vi "TrajectoryGenerate_Make_Quintic_Weighted.vi"(8 "traj_config":T7 {"End Velocity" format="%20.4f"; "StartVelocity" format="%20.4f"; "Max Acceleration" format="%20.4f"; "MaxVelocity" format="%20.4f"}, 11 "WeightedWaypointPOSE":T1[](array[typedef]) {"SCALAR" format="%14.3f"; "ROTATION"."SIN" format="%13.4f"; "ROTATION"."COS" format="%13.4f"; "ROTATION"."VALUE" format="%13.4f"; "TRANSLATION"."Y" format="%14.3f"; "TRANSLATION"."X" format="%14.3f"}) -> (0 "error out":errorcluster, 3 "TRAJECTORY":T4 {"States"."POSE"."ROTATION"."SIN" format="%13.4f"; "States"."POSE"."ROTATION"."COS" format="%13.4f"; "States"."POSE"."ROTATION"."VALUE" format="%13.4f"; "States"."POSE"."TRANSLATION"."Y" format="%14.3f"; "States"."POSE"."TRANSLATION"."X" format="%14.3f"; "TotalTImeSecs" format="%20.3f"})   [LabVIEW 2019, in "Trajectory_Library.lvlib"]
doc: "Generates a trajectory from the given weighted waypoints and config. This method uses quintic hermite splines -- therefore, all points must be represented by Pose2d objects. Continuous curvature is guaranteed in this method.\n\nParameters:\n - WeightedWaypointPose - Array of weighted waypoints .\n - Trajectory Config - The configuration for the trajectory.\n\nReturns:\n - Trajectory -- Created trajectory data structure\n - Error Out - Returned error cluster"
uses:
  Trajectory_Library.lvlib
  TypeDef/TRAJ_CONFIG.ctl
  TypeDef/TRAJECTORY.ctl
  TypeDef/TRAJ_STATE.ctl
  TypeDef/POSE2D.ctl
  TypeDef/TRANSLATION2D.ctl
  TypeDef/ROTATION2D.ctl
  TypeDef/WEIGHTED_WAYPOINT.ctl
  TypeDef/POSEwCURVATURE.ctl
  Conv_Deg_Radians.vi
  Rotation2d_CreateAngle.vi
  Pose2d_TransformBy.vi
  Translation2d_RotateBy.vi
  Translation2d_Plus.vi
  Rotation2d_Plus.vi
  Rotation2d_RotateBy.vi
  Rotation2d_CreateXY.vi
  Util_CalcDist.vi
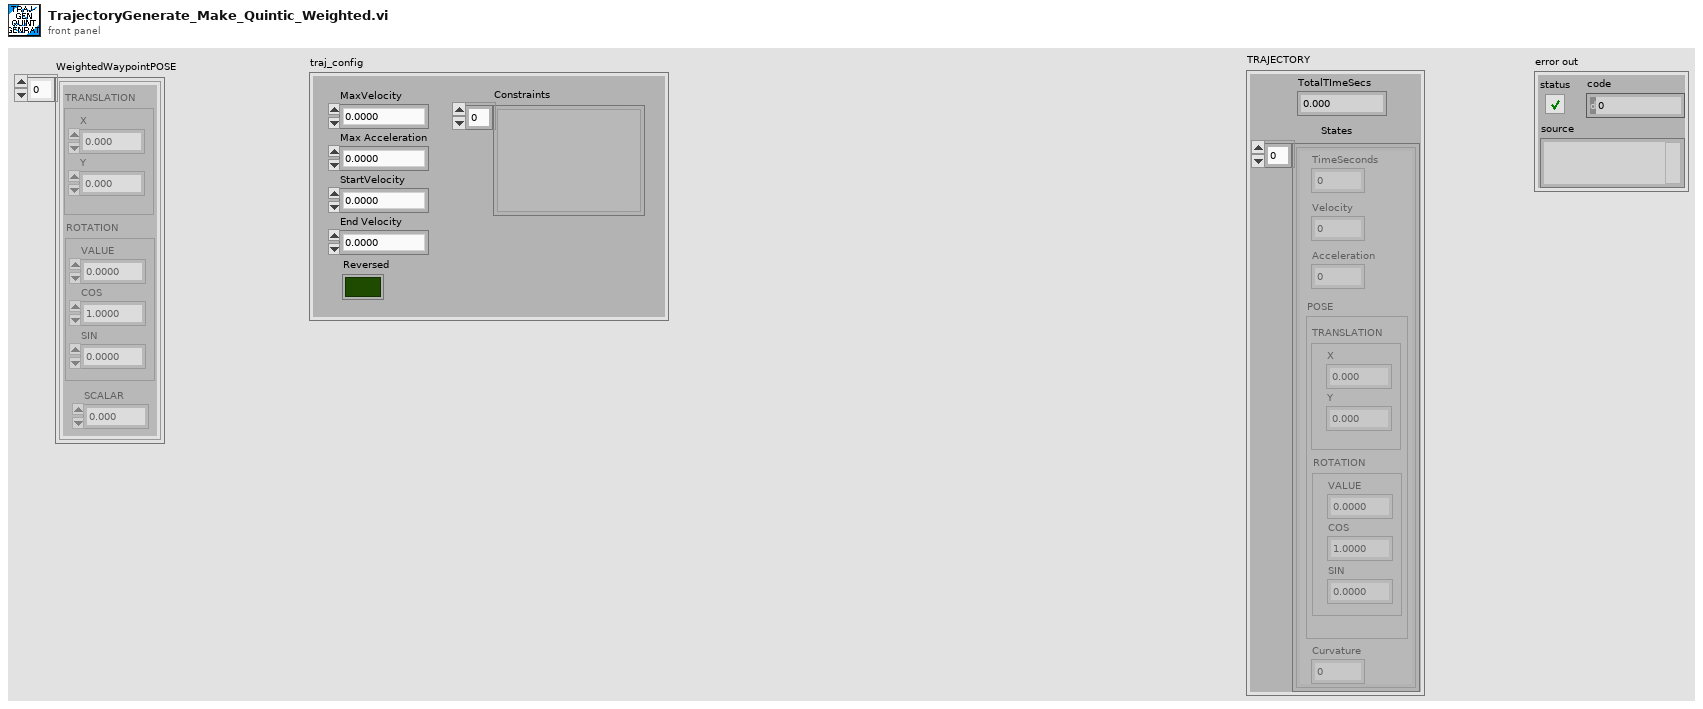
[diagram p1: front panel]
types:
  T1 = typedef "Trajectory_Library.lvlib/WEIGHTED_WAYPOINT.ctl" = cluster{"TRANSLATION":T2, "ROTATION":T3, "SCALAR":dbl}
  T2 = typedef "Trajectory_Library.lvlib/TRANSLATION2D.ctl" = cluster{"X":dbl, "Y":dbl}
  T3 = typedef "Trajectory_Library.lvlib/ROTATION2D.ctl" = cluster{"VALUE":dbl, "COS":dbl, "SIN":dbl}
  T4 = typedef "Trajectory_Library.lvlib/TRAJECTORY.ctl" = cluster{"TotalTImeSecs":dbl, "States":T5[]}
  T5 = typedef "Trajectory_Library.lvlib/TRAJ_STATE.ctl" = cluster{"TimeSeconds":dbl, "Velocity":dbl, "Acceleration":dbl, "POSE":T6, "Curvature":dbl}
  T6 = typedef "Trajectory_Library.lvlib/POSE2D.ctl" = cluster{"TRANSLATION":T2, "ROTATION":T3}
  T7 = typedef "Trajectory_Library.lvlib/TRAJ_CONFIG.ctl" = cluster{"MaxVelocity":dbl, "Max Acceleration":dbl, "StartVelocity":dbl, "End Velocity":dbl, "Reversed":bool, "Constraints":variant[]}
  T8 = typedef "Trajectory_Library.lvlib/TRANSFORM2D.ctl" = cluster{"TRANSLATION":T2, "ROTATION":T3, "xF":bool}
  T9 = typedef "Trajectory_Library.lvlib/SPLINE.ctl" = cluster{"Degree":i32, "Coefficients":T10}
  T10 = typedef "NI_Matrix.lvlib/RealMatrix.ctl" = dbl[][]
  T11 = typedef "Trajectory_Library.lvlib/POSEwCURVATURE.ctl" = cluster{"CURVATURE":dbl, "POSE":T6}
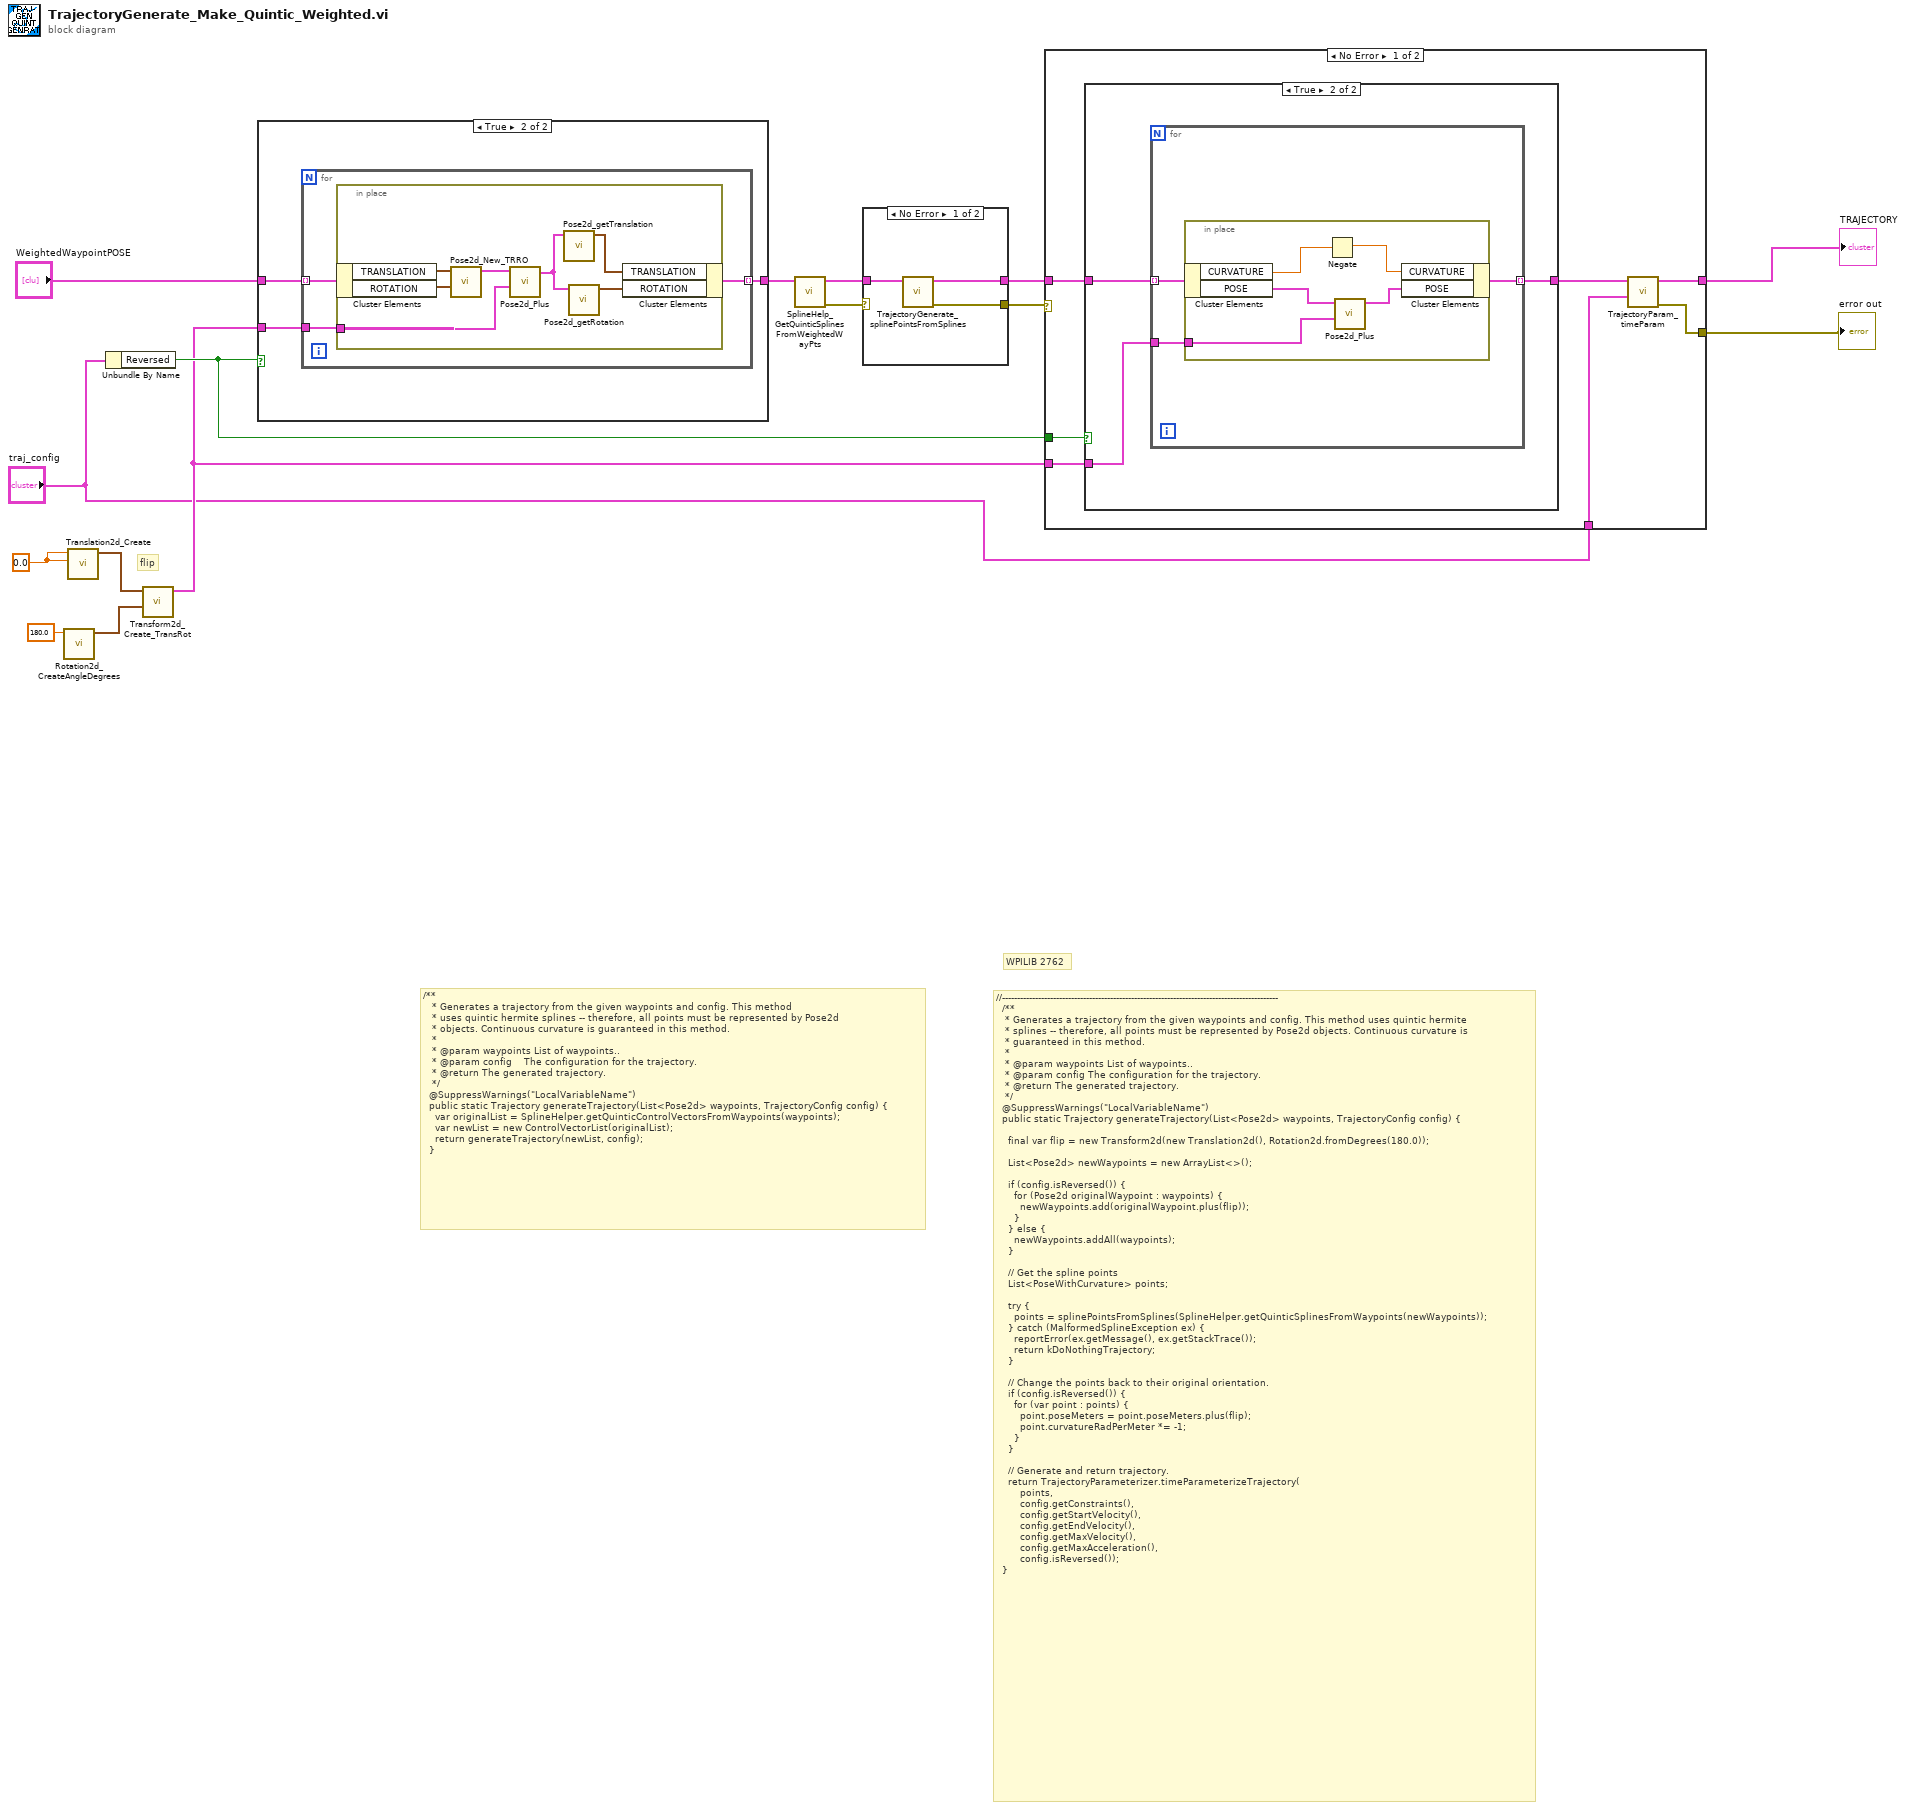
[diagram p0: block diagram]
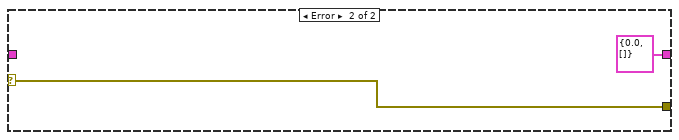
[diagram p3: hidden frame]
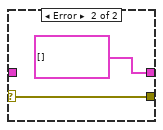
[diagram p4: hidden frame]
diagram:
  w13 = 0.0 ("X")
  # "flip"
  # "WPILIB 2762"
  # "//--------------------------------------------------------------------------------------------\n  /**\n   * Generates a trajectory from the given waypoints and config. This method uses quintic hermite\n   * splines -- therefore, all points must be represented by Pose2d objects. Continuous curvature is\n   * guaranteed in this method.\n   *\n   * @param waypoints List of waypoints..\n   * @param config The configuration for the trajectory.\n   * @return The generated trajectory.\n   */\n  @SuppressWarnings(\"LocalVariableName\")\n  public static Trajectory generateTrajectory(List<Pose2d> waypoints, TrajectoryConfig config) {\n\n    final var flip = new Transform2d(new Translation2d(), Rotation2d.fromDegrees(180.0));\n\n    List<Pose2d> newWaypoints = new ArrayList<>();\n\n    if (config.isReversed()) {\n      for (Pose2d originalWaypoint : waypoints) {\n        newWaypoints.add(originalWaypoint.plus(flip));\n      }\n    } else {\n      newWaypoints.addAll(waypoints);\n    }\n\n    // Get the spline points\n    List<PoseWithCurvature> points;\n\n    try {\n      points = splinePointsFromSplines(SplineHelper.getQuinticSplinesFromWaypoints(newWaypoints));\n    } catch (MalformedSplineException ex) {\n      reportError(ex.getMessage(), ex.getStackTrace());\n      return kDoNothingTrajectory;\n    }\n\n    // Change the points back to their original orientation.\n    if (config.isReversed()) {\n      for (var point : points) {\n        point.poseMeters = point.poseMeters.plus(flip);\n        point.curvatureRadPerMeter *= -1;\n      }\n    }\n\n    // Generate and return trajectory.\n    return TrajectoryParameterizer.timeParameterizeTrajectory(\n        points,\n        config.getConstraints(),\n        config.getStartVelocity(),\n        config.getEndVelocity(),\n        config.getMaxVelocity(),\n        config.getMaxAcceleration(),\n        config.isReversed());\n  }"
  # "/**\n   * Generates a trajectory from the given waypoints and config. This method\n   * uses quintic hermite splines -- therefore, all points must be represented by Pose2d\n   * objects. Continuous curvature is guaranteed in this method.\n   *\n   * @param waypoints List of waypoints..\n   * @param config    The configuration for the trajectory.\n   * @return The generated trajectory.\n   */\n  @SuppressWarnings(\"LocalVariableName\")\n  public static Trajectory generateTrajectory(List<Pose2d> waypoints, TrajectoryConfig config) {\n    var originalList = SplineHelper.getQuinticControlVectorsFromWaypoints(waypoints);\n    var newList = new ControlVectorList(originalList);\n    return generateTrajectory(newList, config);\n  }"
  n1 = call "Rotation2d_CreateAngleDegrees.vi"("Angle_Degrees"=180.0) -> ("ROTATION"=w15:T3)  [unwired: 10 in]
  n2 = call "Translation2d_Create.vi"("Y"=w13, "X"=w13) -> ("TRANSLATION"=w12:T2)  [unwired: 9 in]
  n3 = Unbundle By Name("traj_config") -> ("Reversed"=w6:bool)
  n4 = call "Transform2d_Create_TransRot.vi"("ROTATION"=w15, "TRANSLATION"=w12) -> ("TRANSFORM"=w4:T8)  [unwired: 9 in]
  n5 = case shown="True" w6 {
    tunnel: "WeightedWaypointPOSE" -> [w16 w19]
    tunnel: w4 -> [_ w18]
    tunnel: [w16 w17] -> w10
    frame False {
    }
    frame True {
      n6 = for {
        tunnel: w19 -> [w21] mode=indexing
        tunnel: w18 -> [w22]
        tunnel: [w20] -> w17 mode=indexing
        n7 = in-place {
          in-place-border: w22 -> [w26]
          n8 = in-place-cluster #1(w21) -> ("TRANSLATION"=w29:T2, "ROTATION"=w28:T3)
          n9 = call "Pose2d_New_TRRO.vi"("ROTATION"=w28, "TRANSLATION"=w29) -> ("outPOSE"=w27:T6)  [unwired: 9 in]
          n10 = call "Pose2d_Plus.vi"("other TRANSFORM"=w26, "in POSE"=w27) -> ("out POSE"=w23:T6)  [unwired: 9 in]
          n11 = call "Pose2d_getTranslation.vi"("in POSE"=w23) -> ("outTRANSLATION"=w24:T2)  [unwired: 10 in]
          n12 = call "Pose2d_getRotation.vi"("in POSE"=w23) -> ("out ROTATION"=w25:T3)  [unwired: 10 in]
          n13 = in-place-cluster #1("TRANSLATION"=w24, "ROTATION"=w25) -> (w20:T1)
        }
      }
    }
  }
  n14 = call "SplineHelp_GetQuinticSplinesFromWeightedWayPts.vi"("WeightedWayPoints"=w10) -> ("out Error"=w9:errorcluster, "Splines"=w8:T9[])  [unwired: 9 in]
  n15 = case shown="No Error" w9 {
    selector: w9 -> [_ w34]
    tunnel: w8 -> [w32 _]
    tunnel: [w31 w34] -> w7
    tunnel: [w30 T11[] [] ("ArrayPoseWithCurvature")] -> w5
    frame No Error {
      n16 = call "TrajectoryGenerate_splinePointsFromSplines.vi"("inputSPLINE"=w32) -> ("error out"=w31:errorcluster, "ArrayPoseWithCurvature"=w30:T11[])  [unwired: 9 in]
    }
    frame Error {
    }
  }
  n17 = case shown="No Error" w7 {
    selector: w7 -> [_ w55]
    tunnel: w6 -> [w41 _]
    tunnel: w5 -> [w40 _]
    tunnel: w4 -> [w39 _]
    tunnel: "traj_config" -> [w37 _]
    tunnel: [w36 T4 {"TotalTImeSecs"=0.0, "States"=[]} ("TRAJECTORY")] -> w2
    tunnel: [w35 w55] -> w1
    frame No Error {
      n18 = case shown="True" w41 {
        tunnel: w40 -> [w42 w45]
        tunnel: w39 -> [_ w44]
        tunnel: [w42 w43] -> w38
        frame False {
        }
        frame True {
          n19 = for {
            tunnel: w45 -> [w48] mode=indexing
            tunnel: w44 -> [w47]
            tunnel: [w46] -> w43 mode=indexing
            n20 = in-place {
              in-place-border: w47 -> [w49]
              n21 = in-place-cluster #2(w48) -> ("CURVATURE"=w53:dbl, "POSE"=w52:T6)
              n22 = Negate(x=w53) -> (-x=w50:dbl)
              n23 = call "Pose2d_Plus.vi"("other TRANSFORM"=w49, "in POSE"=w52) -> ("out POSE"=w51:T6)  [unwired: 9 in]
              n24 = in-place-cluster #2("CURVATURE"=w50, "POSE"=w51) -> (w46:T11)
            }
          }
        }
      }
      n25 = call "TrajectoryParam_timeParam.vi"("TRAJECTORY_CONFIG"=w37, "points"=w38) -> ("error out"=w35:errorcluster, "TRAJECTORY"=w36:T4)  [unwired: 8 in]
    }
    frame Error {
    }
  }
  "TRAJECTORY" <- w2
  "error out" <- w1
